vi "AIAverager4Ch.vi"(11 "Array in":dbl[](array[numeric])) -> (3 "Array out":dbl[](array[numeric]))   [LabVIEW 2018, in "Inputs.lvlib"]
uses:
  Inputs.lvlib
  <vilib>/ptbypt/NI_PtbyPt.lvlib
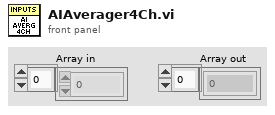
[diagram p1: front panel]
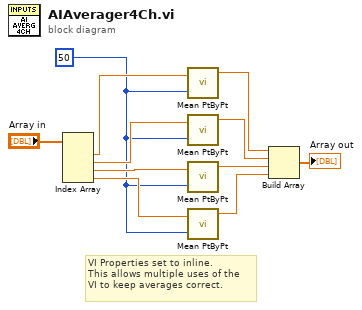
[diagram p0: block diagram]
diagram:
  w3 = 50 ("sample length")
  # "VI Properties set to inline. \nThis allows multiple uses of the \nVI to keep averages correct."
  n1 = Index Array(array="Array in") -> (element #1=w8:dbl, element #2=w9:dbl, element #3=w10:dbl, element #4=w11:dbl)  [unwired: 4 in]
  n2 = call <vilib>:"Mean PtByPt.vi"("x"=w8, "sample length"=w3) -> ("mean"=w2:dbl)  [unwired: 2 in, 1 out]
  n3 = call <vilib>:"Mean PtByPt.vi"("x"=w9, "sample length"=w3) -> ("mean"=w4:dbl)  [unwired: 2 in, 1 out]
  n4 = call <vilib>:"Mean PtByPt.vi"("x"=w10, "sample length"=w3) -> ("mean"=w5:dbl)  [unwired: 2 in, 1 out]
  n5 = call <vilib>:"Mean PtByPt.vi"("x"=w11, "sample length"=w3) -> ("mean"=w6:dbl)  [unwired: 2 in, 1 out]
  n6 = Build Array(w2, w4, w5, w6) -> (→"Array out":dbl[])
